vi "N-Wait.vi"(8 "error in":errorcluster, 9 "timeout in ms (-1)":i32, 11 "Q Name":string) -> (0 "error out":errorcluster, 1 "timed out?":bool, 2 "Waveform":waveform(dbl)[](array[waveform]))   [LabVIEW 2016]
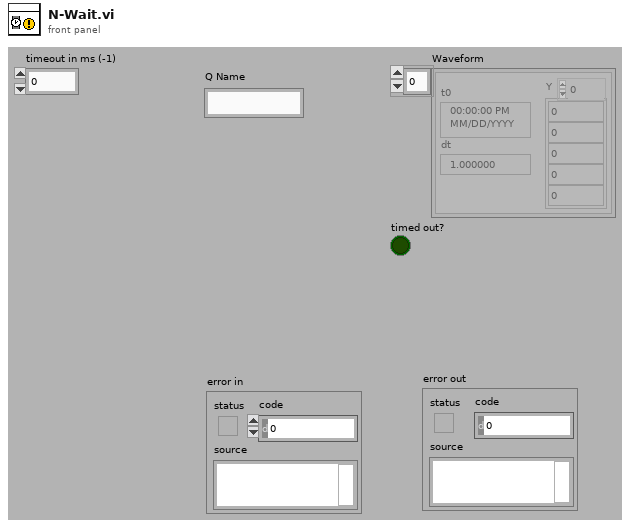
[diagram p1: front panel]
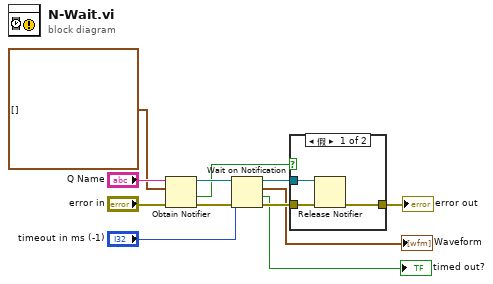
[diagram p0: block diagram]
diagram:
  n1 = Obtain Notifier(name (unnamed)="Q Name", notification data type=waveform(dbl)[] [] ("Waveform"), error in (no error)="error in") -> (notifier out=w11:refnum<notifier>, created new?=w9:bool, error out=w4:errorcluster)  [unwired: 1 in]
  n2 = Wait on Notification(notifier=w11, timeout in ms (-1)="timeout in ms (-1)", error in (no error)=w4) -> (notifier out=w8:refnum<notifier>, notification=→"Waveform":waveform(dbl)[], timed out?=→"timed out?":bool, error out=w7:errorcluster)  [unwired: 1 in]
  n3 = case shown="假" w9 {
    tunnel: w8 -> [w15 _]
    tunnel: w7 -> [w14 w16]
    tunnel: [w13 w16] -> w6
    frame False {
      n4 = Release Notifier(notifier=w15, error in (no error)=w14) -> (error out=w13:errorcluster)  [unwired: 1 in, 2 out]
    }
    frame True {
    }
  }
  "error out" <- w6
